vi "Find Workspace sensor cheat.vi"(8 "error in (no error)":errorcluster, 10 "Control In":T2, 11 "Component.lvclass":refnum<class "Component Tray.lvclass">) -> (0 "error out":errorcluster, 1 "Workspace":T1, 2 "Control Out":T2, 3 "Workspace Out":refnum<class "Component Tray.lvclass">)   [LabVIEW 2019, in "Component Tray.lvclass"]
uses:
  Component Tray.lvclass
  Workspace.ctl
  Fixture.lvclass
  Controller/Controllers.ctl
  Controller/Controller.lvclass
  Controller/I-O/I-O.lvclass
  Controller/Dispenser/Dispenser.lvclass
  C:/Program Files (x86)/Aerotech/A3200/LabVIEW/2010/Bin/Aerotech.A3200.dll
  Program Files (x86)/Aerotech/A3200/LabVIEW/2010/Bin/Aerotech.A3200.dll
panel:
  out "Workspace 2":T1
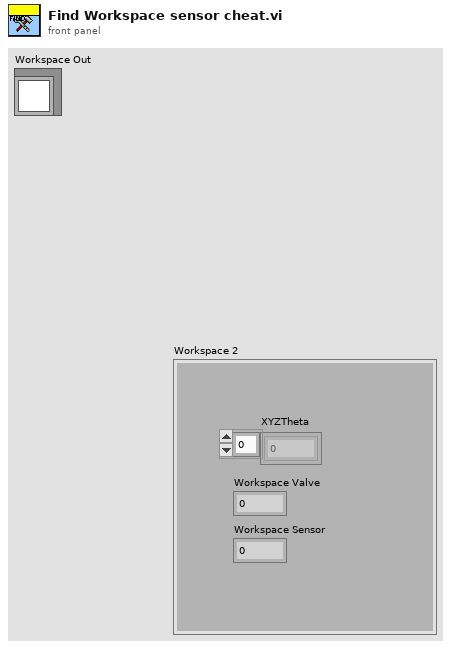
[diagram p1: front panel]
types:
  T1 = typedef "Fixture.lvclass/Workspace.ctl" = cluster{"XYZTheta":dbl[], "Workspace Valve":i32, "Workspace Sensor":i32}
  T2 = typedef "Controller.lvclass/Controllers.ctl" = cluster{"I-O.lvclass":refnum<class "I-O.lvclass">, "Dispenser.lvclass":refnum<class "Dispenser.lvclass">, "Gantry":refnum<k24>}
  T3 = typedef "File Paths.ctl" = cluster{"Glue Pattern Folder":path, "Carrier Tray Folder":path, "Pick Up Tool Fixture Folder":path, "Components Folder":path, "Bellows Tool Offset.txt":path, "Pick Up Tool Offset.txt":path, "Dispense Tip Offset.txt":path, "Log Files":path}
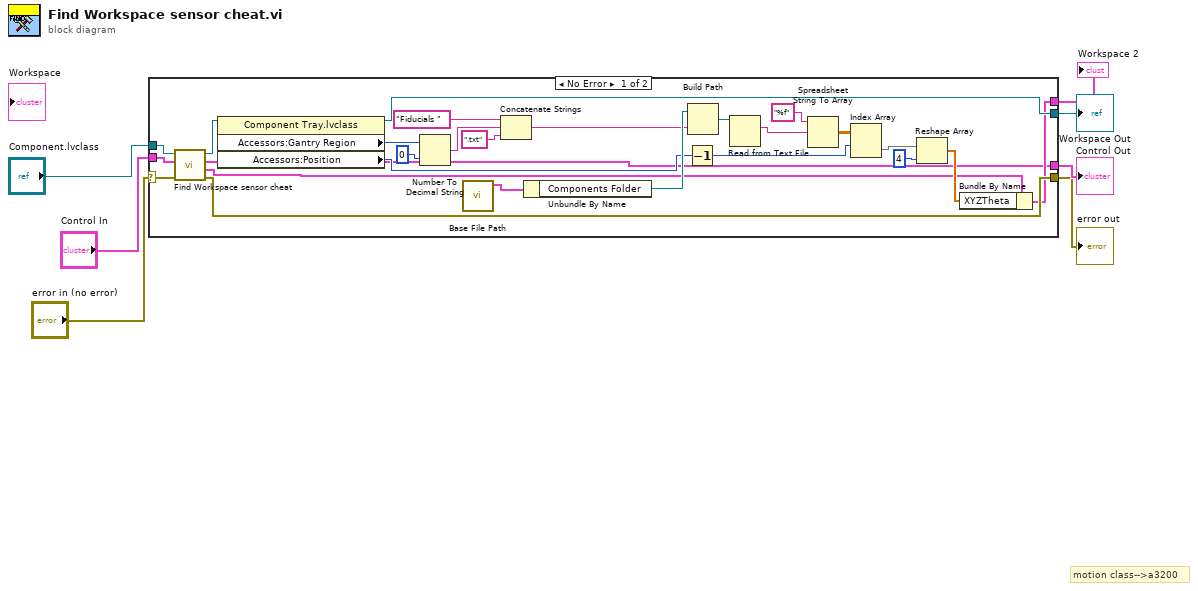
[diagram p0: block diagram]
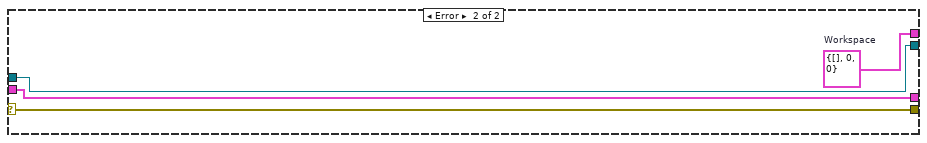
[diagram p2: hidden frame]
diagram:
  # "motion class-->a3200"
  n1 = case shown="No Error" "error in (no error)" {
    selector: "error in (no error)" -> [w32 w37]
    tunnel: [w8 w36] -> w7
    tunnel: [w33 w37] -> w6
    tunnel: [w9 w35] -> w1
    tunnel: "Control In" -> [w31 w36]
    tunnel: [w28 w34] -> w3
    tunnel: "Component.lvclass" -> [w30 w34]
    frame No Error {
      n2 = call-parent "Find Workspace sensor cheat.vi"("Error In"=w32, "Control In"=w31, "Workspace In"=w30) -> ("Error Out"=w33:errorcluster, 1:"Workspace Out"=w10:T1, "Control Out"=w8:T2, 3:"Workspace Out"=w29:refnum<class "Component Tray.lvclass">)  [unwired: 5 in]
      n3 = property class="Component Tray.lvclass"(reference=w29) -> (reference out=w28:refnum<class "Component Tray.lvclass">, "Accessors:Gantry Region"=w11:i32, "Accessors:Position"=w12:i32)  [unwired: 1 in, 1 out]
      n4 = Number To Decimal String(number=w11, width (-)=i16 0) -> (decimal integer string=w25:string)
      n5 = call "Base File Path.vi"() -> ("Paths Out"=w27:T3)  [unwired: 11 in]
      n6 = Concatenate Strings("Fiducials " ("string"), w25, ".txt") -> (w22:string)
      n7 = Unbundle By Name(w27) -> ("Components Folder"=w23:path)
      n8 = Decrement(x=w12) -> (x-1=w14:i32)
      n9 = Build Path(base path=w23, name or relative path=w22) -> (appended path=w21:path)
      n10 = Read from Text File(file (use dialog)=w21) -> (text=w20:string)  [unwired: 3 in, 3 out]
      n11 = Spreadsheet String To Array(format string="%f", spreadsheet string=w20) -> (array=w18:dbl[][])  [unwired: 2 in]
      n12 = Index Array(array=w18, index (row)=w14) -> (element=w17:dbl[])  [unwired: 1 in]
      n13 = Reshape Array(w17, 4 ("dimension size")) -> (w15:dbl[])
      n14 = Bundle By Name(cluster=w10, "XYZTheta"=w15) -> (w9:T1)
    }
    frame Error {
      w35 = T1 {"XYZTheta"=[], "Workspace Valve"=0, "Workspace Sensor"=0}  # Workspace
    }
  }
  "error out" <- w6
  "Control Out" <- w7
  "Workspace Out" <- w3
  "Workspace 2" <- w1
